vi "DQMH_API_Parse Project for DQMH Modules.vi"(8 "error in (no error)":errorcluster, 10 "Allowable Module Type":T1(ring), 11 "Project (unwired: Active Project)":refnum<vi>) -> (0 "error out":errorcluster, 1 "Any Dirty Modules?":bool, 2 "My Computer":refnum<vi>, 3 "DQMH Modules":T2(array[cluster]), 4 "Any Locked Modules?":bool, 5 "project owning folder":path, 6 "All Libraries in Project":string[](array[string]))   [LabVIEW 2016]
doc: "_____\nCreated using Delacor QMH Event Scripter 5.0.0.106."
uses:
  project/Delacor/DQMH/_DQMH New Event/DQMH New Event.lvlib
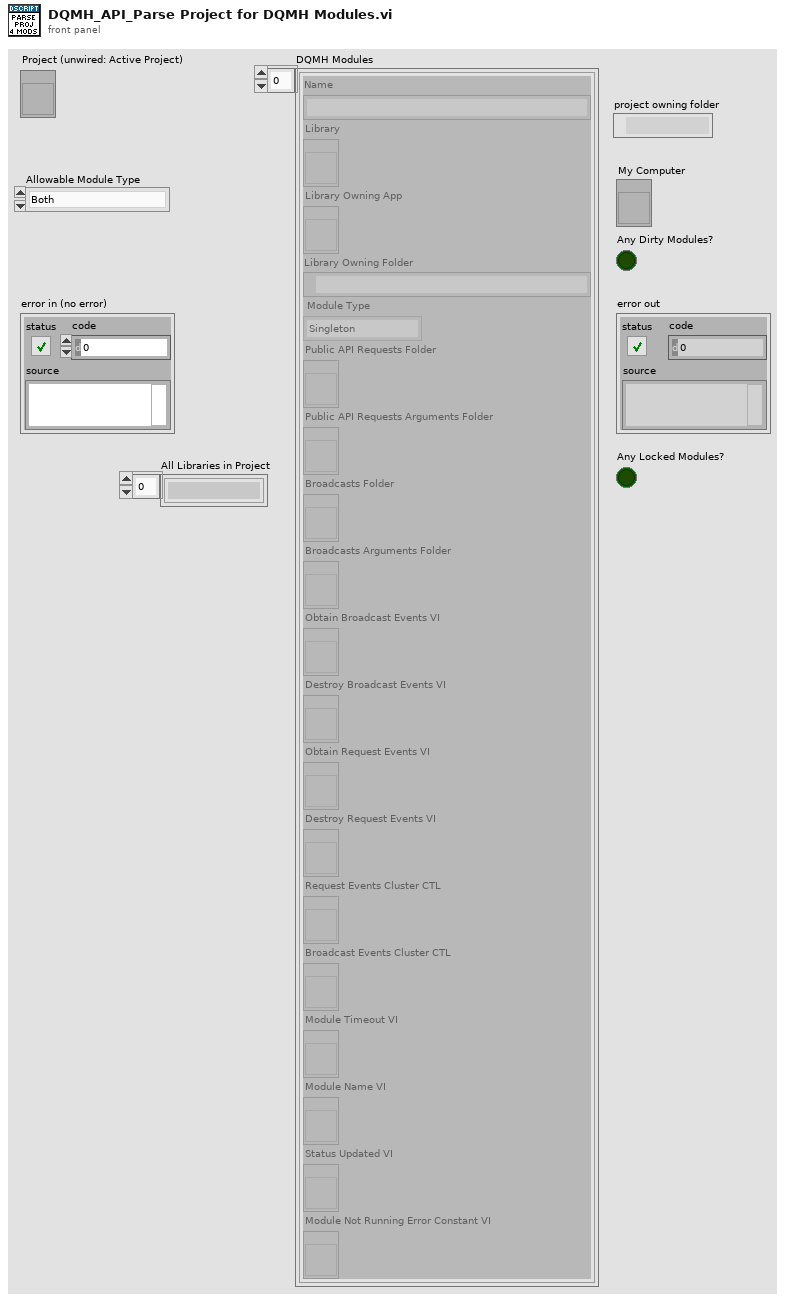
[diagram p1: front panel]
types:
  T1 = enum16{"Both", "Singleton Only", "Cloneable Only"}
  T2 = cluster{"Name":string, "Library":refnum<vi>, "Library Owning App":refnum<vi>, "Library Owning Folder":path, "Module Type":enum16{"Singleton", "Cloneable"}, "Public API Requests Folder":refnum<vi>, "Public API Requests Arguments Folder":refnum<vi>, "Broadcasts Folder":refnum<vi>, "Broadcasts Arguments Folder":refnum<vi>, "Obtain Broadcast Events VI":refnum<vi>, "Destroy Broadcast Events VI":refnum<vi>, "Obtain Request Events VI":refnum<vi>, "Destroy Request Events VI":refnum<vi>, "Request Events Cluster CTL":refnum<vi>, "Broadcast Events Cluster CTL":refnum<vi>, "Module Timeout VI":refnum<vi>, "Module Name VI":refnum<vi>, "Status Updated VI":refnum<vi>, "Module Not Running Error Constant VI":refnum<vi>}[]
  T3 = typedef "DQMH New Event.lvlib/Module Info--cluster.ctl" = cluster{"Name":string, "Library":refnum<vi>, "Library Owning App":refnum<vi>, "Library Owning Folder":path, "Module Type":T4, "Public API Requests Folder":refnum<vi>, "Public API Requests Arguments Folder":refnum<vi>, "Broadcasts Folder":refnum<vi>, "Broadcasts Arguments Folder":refnum<vi>, "Obtain Broadcast Events VI":refnum<vi>, "Destroy Broadcast Events VI":refnum<vi>, "Obtain Request Events VI":refnum<vi>, "Destroy Request Events VI":refnum<vi>, "Request Events Cluster CTL":refnum<vi>, "Broadcast Events Cluster CTL":refnum<vi>, "Module Timeout VI":refnum<vi>, "Module Name VI":refnum<vi>, "Status Updated VI":refnum<vi>, "Module Not Running Error Constant VI":refnum<vi>}
  T4 = typedef "DQMH New Event.lvlib/Module Type--enum.ctl" = enum16{"Singleton", "Cloneable"}
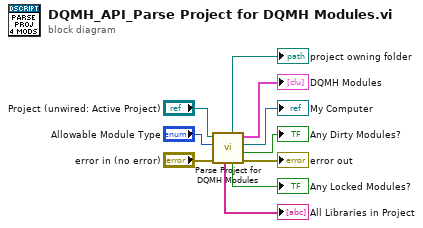
[diagram p0: block diagram]
diagram:
  n1 = call "Parse Project for DQMH Modules.vi"("error in (no error)"="error in (no error)", "Allowable Module Type"="Allowable Module Type", "Project (unwired: Active Project)"="Project (unwired: Active Project)") -> ("error out"=→"error out":errorcluster, "Any Dirty Modules?"=→"Any Dirty Modules?":bool, "My Computer"=→"My Computer":refnum<vi>, "DQMH Modules"=→"DQMH Modules":T3[], "Any Locked Modules?"=→"Any Locked Modules?":bool, "project owning folder"=→"project owning folder":path, "All Libraries in Project"=→"All Libraries in Project":string[])  [unwired: 2 in]
